vi "AWG VHi&VLo&AmpGain to Gain&Offset.vi"(9 "AmpGain":i32, 10 "VLo":dbl, 11 "VHi":dbl) -> (2 "Offset":dbl, 3 "Gain":dbl)   [LabVIEW 2013]
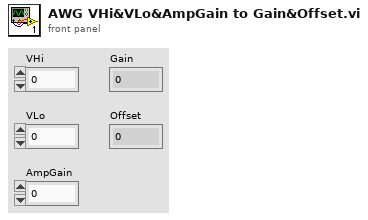
[diagram p1: front panel]
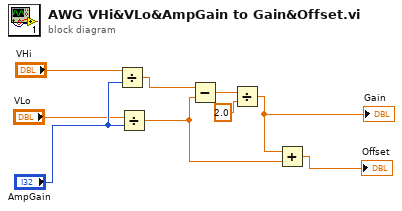
[diagram p0: block diagram]
diagram:
  n1 = Divide(x="VHi", y="AmpGain") -> (x/y=w6:dbl)
  n2 = Divide(x="VLo", y="AmpGain") -> (x/y=w9:dbl)
  n3 = Subtract(x=w6, y=w9) -> (x-y=w2:dbl)
  n4 = Divide(x=w2, y=2.0) -> (x/y=w8:dbl)
  "Gain" <- w8
  n5 = Add(x=w8, y=w9) -> (x+y=→"Offset":dbl)
